vi "Init Switch - Voltage Mode.vi"(8 "error in (no error)":errorcluster, 9 "Switch -> DMM Trigger":u16, 10 "DMM -> Switch Trigger":u16, 11 "Switch Device in":refnum<k15>) -> (0 "error out":errorcluster, 3 "Switch Device out":refnum<k15>)   [LabVIEW 2011, in "Switch-DMM Custom Device.lvlib"]
uses:
  Switch-DMM Custom Device.lvlib
  <instrlib>/niSwitch/niSwitch.LLB/niSwitch Scan Advanced Output.ctl
  <instrlib>/niSwitch/niSwitch.LLB/niSwitch Scan Mode.ctl
  <instrlib>/niSwitch/niSwitch.LLB/niSwitch Trigger Input.ctl
  <instrlib>/niSwitch/niSwitch.LLB/niSwitch Connect Channels (Single).vi
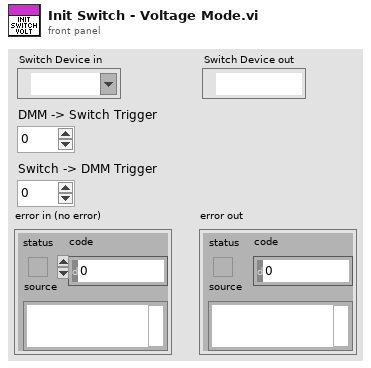
[diagram p1: front panel]
types:
  T1 = typedef "niSwitch Scan Advanced Output.ctl" = enum16{"None", "External", "TTL0", "TTL1", "TTL2", "TTL3", "TTL4", "TTL5", "TTL6", "TTL7", "ECL0", "ECL1", "PXI Star", "Rear Connector", "Front Connector", "Rear Connector Module 1", "Rear Connector Module 2", "Rear Connector Module 3", "Rear Connector Module 4", "Rear Connector Module 5", "Rear Connector Module 6", "Rear Connector Module 7", "Rear Connector Module 8", "Rear Connector Module 9", "Rear Connector Module 10", "Rear Connector Module 11", "Rear Connector Module 12", "Front Connector Module 1", "Front Connector Module 2", "Front Connector Module 3", "Front Connector Module 4", "Front Connector Module 5", "Front Connector Module 6", "Front Connector Module 7", "Front Connector Module 8", "Front Connector Module 9", "Front Connector Module 10", "Front Connector Module 11", "Front Connector Module 12"}
  T2 = typedef "niSwitch Scan Mode.ctl" = enum16{"No Action", "Break Before Make", "Break After Make"}
  T3 = typedef "niSwitch Trigger Input.ctl" = enum16{"Immediate", "External", "TTL0", "TTL1", "TTL2", "TTL3", "TTL4", "TTL5", "TTL6", "TTL7", "ECL0", "ECL1", "PXI Star", "Software Trigger Function", "Rear Connector", "Front Connector", "Rear Connector of Module 1", "Rear Connector of Module 2", "Rear Connector of Module 3", "Rear Connector of Module 4", "Rear Connector of Module 5", "Rear Connector of Module 6", "Rear Connector of Module 7", "Rear Connector of Module 8", "Rear Connector of Module 9", "Rear Connector of Module 10", "Rear Connector of Module 11", "Rear Connector of Module 12", "Front Connector of Module 1", "Front Connector of Module 2", "Front Connector of Module 3", "Front Connector of Module 4", "Front Connector of Module 5", "Front Connector of Module 6", "Front Connector of Module 7", "Front Connector of Module 8", "Front Connector of Module 9", "Front Connector of Module 10", "Front Connector of Module 11", "Front Connector of Module 12"}
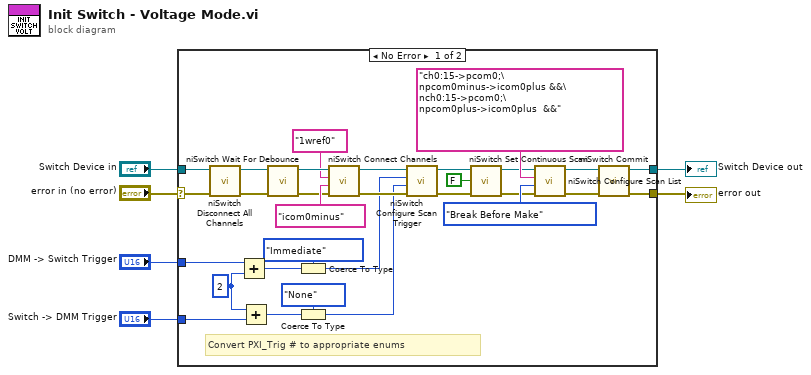
[diagram p0: block diagram]
diagram:
  n1 = case shown="No Error" "error in (no error)" {
    selector: "error in (no error)" -> [w7 w37]
    tunnel: [w36 w37] -> w1
    tunnel: [w35 w38] -> w2
    tunnel: "Switch Device in" -> [w17 w38]
    tunnel: "DMM -> Switch Trigger" -> [w16 _]
    tunnel: "Switch -> DMM Trigger" -> [w14 _]
    frame No Error {
      w15 = u16 2 ("y")
      # "Convert PXI_Trig # to appropriate enums"
      n2 = call <instrlib>:"niSwitch Disconnect All Channels.vi"("error in (no error)"=w7, "instrument handle"=w17) -> ("error out"=w19:errorcluster, "instrument handle out"=w20:refnum<k15>)  [unwired: 8 in]
      n3 = Add(x=w16, y=w15) -> (x+y=w13:u16)
      n4 = Add(x=w15, y=w14) -> (x+y=w12:u16)
      n5 = call <instrlib>:"niSwitch Wait For Debounce.vi"("error in (no error)"=w19, "instrument handle"=w20) -> ("error out"=w22:errorcluster, "instrument handle out"=w21:refnum<k15>)  [unwired: 8 in]
      n6 = Coerce To Type(0:w13, 1:niSwitch_Trigger_Input."Immediate" ("trigger input (External)")) -> (2:w10:T3)
      n7 = Coerce To Type(0:w12, 1:niSwitch_Scan_Advanced_Output."None" ("scan advanced output (External)")) -> (2:w8:T1)
      n8 = call-poly <instrlib>:"niSwitch Connect Channels.vi"("error in (no error)"=w22, "channel 2"="icom0minus", "channel 1"="1wref0", "instrument handle"=w21) -> ("error out"=w31:errorcluster, "instrument handle out"=w30:refnum<k15>)  [unwired: 6 in]
      n9 = call <instrlib>:"niSwitch Configure Scan Trigger.vi"("error in (no error)"=w31, "scan advanced output (External)"=w8, "trigger input (External)"=w10, "instrument handle"=w30) -> ("error out"=w28:errorcluster, "instrument handle out"=w29:refnum<k15>)  [unwired: 1 in, 5 out]
      n10 = call <instrlib>:"niSwitch Set Continuous Scan.vi"("error in (no error)"=w28, "continuous scan (False)"=FALSE, "instrument handle"=w29) -> ("error out"=w26:errorcluster, "instrument handle out"=w27:refnum<k15>)  [unwired: 7 out]
      n11 = call <instrlib>:"niSwitch Configure Scan List.vi"("error in (no error)"=w26, "scan mode (Break Before Make)"=niSwitch_Scan_Mode."Break Before Make", "scan list"="ch0:15->pcom0;\npcom0minus->icom0plus &&\nch0:15->pcom0;\npcom0plus->icom0plus  &&", "instrument handle"=w27) -> ("error out"=w25:errorcluster, "instrument handle out"=w24:refnum<k15>)  [unwired: 6 out]
      n12 = call <instrlib>:"niSwitch Commit.vi"("error in (no error)"=w25, "instrument handle"=w24) -> ("error out"=w36:errorcluster, "instrument handle out"=w35:refnum<k15>)  [unwired: 8 out]
    }
    frame Error {
    }
  }
  "error out" <- w1
  "Switch Device out" <- w2
